vi "kinematic_center_constraint.vi"(9 "Goal tip pos":sgl[](array[numeric]), 10 "Goal pose (handle basis) in":T12 format="%#_4g", 11 "Parameters":T1={"Stimulus"={"Type"=enum."Off", "Phase"=0.0, "Amplitude"=[], "Injection point"=enum."Total pose", "Closed loop"=FALSE, "Offset"=[], "Tip -> world"=FALSE, "Frequency"=0.0, "Length"=0.0}, "Goal Filter A"={"Speedup max"=0.0, "Speedup thresh"=0.0, "Speedup nonlin"=0.0, "Filters"=[]}, "Mode controls"={"Hold"=FALSE, "Cancellation"=FALSE, "Goal filter"=FALSE, "Trigger"=FALSE}, "Manipulator type"=enum."Current piezo", "Manipulator calibration"={"Tool offsets"=[[0.0, 0.0, 36200.0]], "Handle light calibration"=[], "Base pivots"=[], "Output pivots"=[], "Length center"=0.0, "Workspace height"=[], "Workspace diameter"=[0.0, 0.0, 36200.0], "Stack travel"=400.0, "Saturation pos"=375.0, "Inverse filters"=[], "Strut length"=0.0}, "Network"={"Remote Host"="", "Send Status"=FALSE, "Send Port"=0, "Recv Commands"=FALSE, "Recv Port"=0}, "Goal Filter B"={"Speedup max"=0.0, "Speedup thresh"=0.0, "Speedup nonlin"=0.0, "Filters"=[]}, "Cancellation"={"KP"={"XY"=0.0, "Rxy"=0.0, "Z"=0.0, "Rz"=0.0}, "KI"=0.0, "KD"={"XY"=0.0, "Rxy"=0.0, "Z"=0.0, "Rz"=0.0}, "Max vel"=20.0, "Max acc"=0.001, "Int error limit"=3.0, "RCM gain"=0.0, "Bypass"=FALSE, "Degraded gain"=0.0}, "Transition time"=0.0, "Estimation"={"Link"={"Measure noise"=[], "Process noise"=[], "Alt process noise"=[], "Alt turnoff cycles"=20, "Innovation limit"=[], "Residue threshold"=0.0, "Enable"=FALSE}, "Handle"={"Measure noise"=[], "Process noise"=[], "State limits"=[], "Innovation limit"=[], "Prediction Lookahead"=0.0, "Enable"=FALSE}}} {"Transition time" format="%_3f"; "Cancellation"."Degraded gain" min=0 max=1 step=0.1 format="%#_3p"; "Cancellation"."RCM gain" min=0 max=1 step=0.1 format="%#_3p"; "Cancellation"."KD"."Rz" min=-1 max=1 step=0.01 format="%#_3p"; "Cancellation"."KD"."Rxy" min=-1 max=1 step=0.01 format="%#_3p"; "Cancellation"."KD"."Z" min=-1 max=1 step=0.01 format="%#_3p"; "Cancellation"."KD"."XY" min=-1 max=1 step=0.01 format="%#_3p"; "Cancellation"."KI" min=0 max=1 step=0.01 format="%#_3p"; "Cancellation"."KP"."Rz" min=-1 max=1 step=0.01 format="%#_3p"; "Cancellation"."KP"."Rxy" min=-1 max=1 step=0.01 format="%#_3p"; "Cancellation"."KP"."Z" min=-1 max=1 step=0.01 format="%#_3p"; "Cancellation"."KP"."XY" min=-1 max=1 step=0.01 format="%#_3p"; "Cancellation"."Max acc" format="%#_3p"; "Goal Filter B"."Filters"."V limit range" format="%_3p"; "Goal Filter B"."Filters"."V limit" format="%_3p"; "Goal Filter B"."Filters"."Upper Q" format="%_3f"; "Goal Filter B"."Filters"."Upper Fc" format="%_3p"; "Goal Filter B"."Filters"."Lower Q" format="%_3f"; "Goal Filter B"."Filters"."Scale factor" format="%_3f"; "Goal Filter B"."Filters"."Lower Fc" format="%_3p"; "Goal Filter B"."Speedup nonlin" format="%_3p"; "Goal Filter B"."Speedup thresh" format="%_3p"; "Goal Filter B"."Speedup max" format="%_3p"; "Manipulator calibration"."Strut length" format="%#_4p"; "Manipulator calibration"."Saturation pos" format="%#.1f"; "Manipulator calibration"."Stack travel" format="%#.1f"; "Manipulator calibration"."Length center" format="%#_4p"; "Manipulator calibration"."Output pivots" format="%#_6f"; "Manipulator calibration"."Base pivots" format="%#_6f"; "Manipulator calibration"."Handle light calibration" format="%#.1f"; "Goal Filter A"."Filters"."V limit range" format="%_3p"; "Goal Filter A"."Filters"."V limit" format="%_3p"; "Goal Filter A"."Filters"."Upper Q" format="%_3f"; "Goal Filter A"."Filters"."Upper Fc" format="%_3p"; "Goal Filter A"."Filters"."Lower Q" format="%_3f"; "Goal Filter A"."Filters"."Scale factor" format="%_3f"; "Goal Filter A"."Filters"."Lower Fc" format="%_3p"; "Goal Filter A"."Speedup nonlin" format="%_3p"; "Goal Filter A"."Speedup thresh" format="%_3p"; "Goal Filter A"."Speedup max" format="%_3p"; "Stimulus"."Length" min=0.0 max=100.0 step=100.0 format="%#_4p"; "Stimulus"."Frequency" min=0.0 step=100.0 format="%#_4g"; "Stimulus"."Offset" format="%#_3p"; "Stimulus"."Amplitude" format="%#_3p"; "Stimulus"."Phase" min=-180.0 max=360.0 step=100.0 format="%#.2f"}) -> (0 "Saturation":bool[](array[boolean]), 3 "Goal pose (handle basis) out":T12 format="%#_4g", 4 "Clip point":sgl[][](array[numeric]))   [LabVIEW 2014]
uses:
  <vilib>/Analysis/Matrix/Datatypes/RealMatrix.ctl
  testing/Micron params.ctl
  testing/stimulus.ctl
  testing/injection_point.ctl
  goal_loop_parms.ctl
  testing/mode_conrols.ctl
  testing/manipulator_cal.ctl
  asap/labview/testing/probe_calibration.ctl
  host/network_params.ctl
  cancellation/sq_control_params.ctl
  cancellation/decoupled_gain.ctl
  cancellation/estimation_controls.ctl
  <vilib>/Analysis/baseanly.llb/A x Vector.vi
  utilities/labview/norm_vec_single.vi
  <vilib>/Analysis/NI_AALBase.lvlib
  <vilib>/Analysis/Matrix/NI_Matrix.lvlib
panel:
  # "Limit goal pose to meet kinematic center workspace.  If neither saturation flag is set, then the output pose is the input.  If only the second flag is set, then the RCM is not met, but the tip (might) be.   If the first is set, then the tip goal is not met."
  # "If saturated, this is the nominal and goal position of the kinematic center after clipping to fit the workspace (handle coordinates.)"
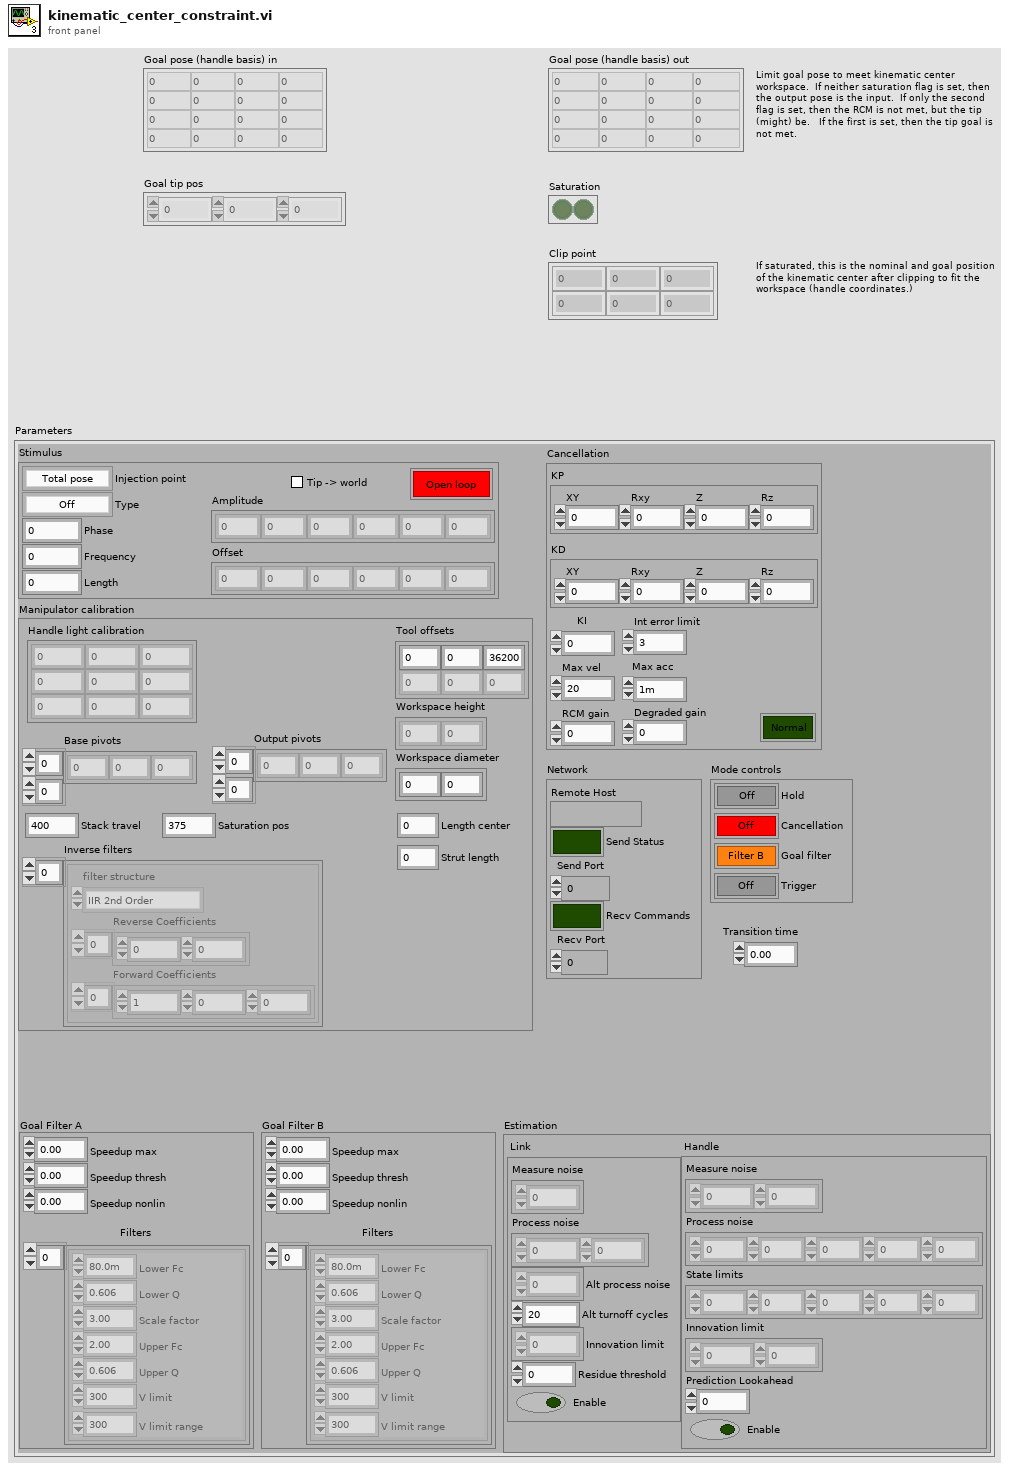
[diagram p1: front panel]
types:
  T1 = typedef "Micron params.ctl" = cluster{"Stimulus":T2, "Goal Filter A":T4, "Mode controls":T5, "Manipulator type":enum16{"Current piezo", "Voltage piezo"}, "Manipulator calibration":T6, "Network":T8, "Goal Filter B":T4, "Cancellation":T9, "Transition time":sgl, "Estimation":T11}
  T2 = typedef "stimulus.ctl" = cluster{"Type":enum16{"Off", "Step", "Sine", "Triangle", "Arbitrary"}, "Phase":dbl, "Amplitude":sgl[], "Injection point":T3, "Closed loop":bool, "Offset":sgl[], "Tip -> world":bool, "Frequency":dbl, "Length":dbl}
  T3 = typedef "injection_point.ctl" = enum16{"Total pose", "V limiter", "Goal ", "Link position", "KF link position", "Inverse kin", "Link goal", "Link error", "Controller", "Output", "Drive", "Light"}
  T4 = typedef "goal_loop_parms.ctl" = cluster{"Speedup max":sgl, "Speedup thresh":sgl, "Speedup nonlin":sgl, "Filters":cluster{"Lower Fc":sgl, "Lower Q":sgl, "Scale factor":sgl, "Upper Fc":sgl, "Upper Q":sgl, "V limit":sgl, "V limit range":sgl}[]}
  T5 = typedef "mode_conrols.ctl" = cluster{"Hold":bool, "Cancellation":bool, "Goal filter":bool, "Trigger":bool}
  T6 = typedef "manipulator_cal.ctl" = cluster{"Tool offsets":sgl[][], "Handle light calibration":T7, "Base pivots":sgl[][], "Output pivots":sgl[][], "Length center":sgl, "Workspace height":sgl[], "Workspace diameter":sgl[], "Stack travel":sgl, "Saturation pos":sgl, "Inverse filters":cluster{"filter structure":enum32{"IIR 2nd Order", "IIR 4th Order"}, "Reverse Coefficients":dbl[], "Forward Coefficients":dbl[]}[], "Strut length":sgl}
  T7 = typedef "probe_calibration.ctl" = sgl[][]
  T8 = typedef "network_params.ctl" = cluster{"Remote Host":string, "Send Status":bool, "Send Port":u16, "Recv Commands":bool, "Recv Port":u16}
  T9 = typedef "sq_control_params.ctl" = cluster{"KP":T10, "KI":sgl, "KD":T10, "Max vel":sgl, "Max acc":sgl, "Int error limit":sgl, "RCM gain":sgl, "Bypass":bool, "Degraded gain":sgl}
  T10 = typedef "decoupled_gain.ctl" = cluster{"XY":sgl, "Rxy":sgl, "Z":sgl, "Rz":sgl}
  T11 = typedef "estimation_controls.ctl" = cluster{"Link":cluster{"Measure noise":dbl[], "Process noise":dbl[], "Alt process noise":dbl[], "Alt turnoff cycles":i32, "Innovation limit":dbl[], "Residue threshold":dbl, "Enable":bool}, "Handle":cluster{"Measure noise":dbl[], "Process noise":dbl[], "State limits":dbl[], "Innovation limit":dbl[], "Prediction Lookahead":sgl, "Enable":bool}}
  T12 = typedef "NI_Matrix.lvlib/RealMatrix.ctl" = dbl[][]
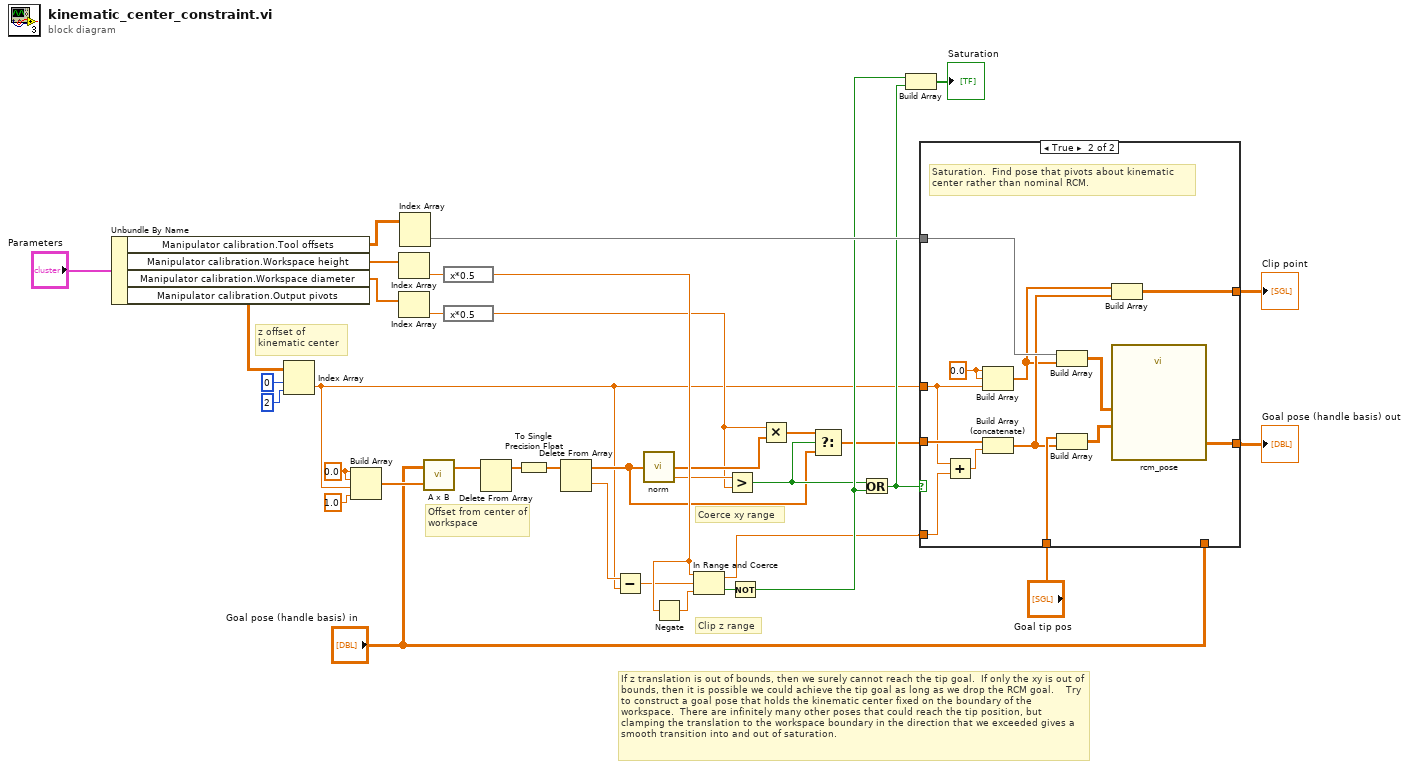
[diagram p0: block diagram]
diagram:
  w34 = sgl 0.0 ("element")
  # "Coerce xy range"
  # "If z translation is out of bounds, then we surely cannot reach the tip goal.  If only the xy is out of bounds, then it is possible we could achieve the tip goal as long as we drop the RCM goal.    Try to construct a goal pose that holds the kinematic center fixed on the boundary of the workspace.  There are infinitely many other poses that could reach the tip position, but clamping the translation to the workspace boundary in the direction that we exceeded gives a smooth transition into and out of saturation."
  # "Clip z range"
  # "Offset from center of workspace"
  # "z offset of \nkinematic center"
  n1 = Unbundle By Name("Parameters") -> ("Manipulator calibration.Tool offsets"=w20:sgl[][], "Manipulator calibration.Workspace height"=w31:sgl[], "Manipulator calibration.Workspace diameter"=w29:sgl[], "Manipulator calibration.Output pivots"=w27:sgl[][])
  n2 = Index Array(array=w27, index (row)=0 ("disabled index (row)"), index (col)=2 ("disabled index (col)")) -> (element=w1:sgl)
  n3 = Build Array(w34, w34, w1, sgl 1.0 ("element")) -> (w36:sgl[])
  n4 = Index Array(array=w31) -> (element=w30:sgl)  [unwired: 1 in]
  n5 = Index Array(array=w29) -> (element=w28:sgl)  [unwired: 1 in]
  n6 = Index Array(array=w20) -> (element=w19:sgl[])  [unwired: 2 in]
  n7 = call-poly <vilib>:"A x B.vi"("Vector"=w36, "A"="Goal pose (handle basis) in") -> ("A x Vector"=w25:dbl[])  [unwired: 1 out]
  n8 = expression code="x*0.5"(w30) -> (w37:sgl)
  n9 = expression code="x*0.5"(w28) -> (w10:sgl)
  n10 = Delete From Array(array=w25) -> (array with subset deleted=w24:dbl[])  [unwired: 2 in, 1 out]
  n11 = To Single Precision Float(number=w24) -> (single precision float=w23:sgl[])
  n12 = Delete From Array(array=w23) -> (deleted portion=w2:sgl, array with subset deleted=w7:sgl[])  [unwired: 2 in]
  n13 = Subtract(x=w2, y=w1) -> (x-y=w3:sgl)
  n14 = call-poly "norm.vi"("vector"=w7) -> ("magnitude"=w21:sgl, "normalized vector"=w11:sgl[])  [unwired: 3 in]
  n15 = Negate(x=w37) -> (-x=w16:sgl)
  n16 = In Range and Coerce(upper limit=w37, x=w3, lower limit=w16) -> (coerced(x)=w13:sgl, In Range?=w15:bool)
  n17 = Greater?(x=w21, y=w10) -> (0:w9:bool)
  n18 = Not(x=w15) -> (.not. x?=w14:bool)
  n19 = Multiply ("Multiply.vi")(x=w10, y=w11) -> (x*y=w8:sgl[])
  n20 = Select(t=w8, s=w9, f=w7) -> (s? t:f=w6:sgl[])
  n21 = Or(x=w9, y=w14) -> (x .or. y?=w17:bool)
  n22 = Build Array(w14, w17) -> (→"Saturation":bool[])
  n23 = case shown="True" w17 {
    tunnel: w1 -> [_ w40]
    tunnel: w19 -> [_ w51]
    tunnel: "Goal tip pos" -> [_ w48]
    tunnel: [w38 w46] -> w5
    tunnel: "Goal pose (handle basis) in" -> [w38 _]
    tunnel: w13 -> [_ w39]
    tunnel: w6 -> [_ w45]
    tunnel: [_ w42] -> w4
    frame False {
    }
    frame True {
      w50 = sgl 0.0 ("Numeric")
      # "Saturation.  Find pose that pivots about kinematic\ncenter rather than nominal RCM."
      n24 = Add(x=w40, y=w39) -> (x+y=w41:sgl)
      n25 = Build Array(w50, w50, w40) -> (w43:sgl[])
      n26 = Build Array (concatenate)(w45, w41) -> (w44:sgl[])
      n27 = Build Array(w51, w43) -> (w49:sgl[][])
      n28 = Build Array(w48, w44) -> (w47:sgl[][])
      n29 = Build Array(w43, w44) -> (w42:sgl[][])
      n30 = call "rcm_pose.vi"("Goal positions"=w47, "Nominal positions"=w49) -> ("Goal pose (handle basis)"=w46:T12)  [unwired: 9 in]
    }
  }
  "Goal pose (handle basis) out" <- w5
  "Clip point" <- w4
